vi "Do.vi"(8 "error in (no error)":errorcluster, 10 "Actor in":refnum<class "Actor.lvclass">, 11 "Self-Addressed Message":refnum<class "Self-Addressed Msg.lvclass">) -> (0 "error out":errorcluster, 2 "Actor out":refnum<class "Actor.lvclass">)   [LabVIEW 2020, in "Actor Framework.lvlib" / "Self-Addressed Msg.lvclass"]
uses:
  Self-Addressed Msg.lvclass
  Self-Addressed Msg.lvclass/Self-Addressed Msg.ctl
  Message/Message.lvclass
  Actor/Actor.lvclass
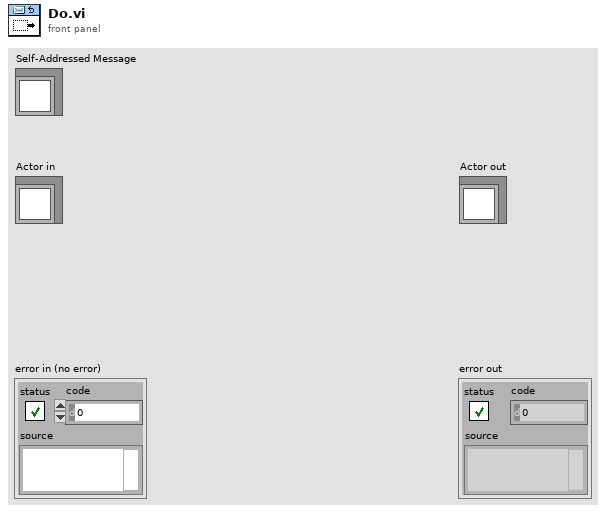
[diagram p1: front panel]
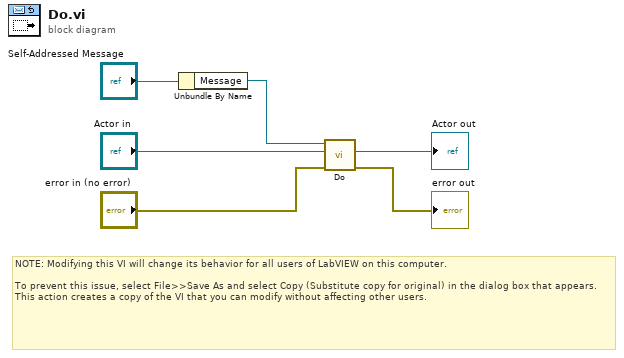
[diagram p0: block diagram]
diagram:
  # "NOTE: Modifying this VI will change its behavior for all users of LabVIEW on this computer.\n\nTo prevent this issue, select File>>Save As and select Copy (Substitute copy for original) in the dialog box that appears. This action creates a copy of the VI that you can modify without affecting other users."
  n1 = Unbundle By Name("Self-Addressed Message") -> ("Message"=w5:refnum<class "Message.lvclass">)
  n2 = call-dynamic "Do.vi"("error in (no error)"="error in (no error)", "Actor in"="Actor in", "Message"=w5) -> ("error out"=→"error out":errorcluster, "Actor out"=→"Actor out":refnum<class "Actor.lvclass">)  [unwired: 7 in]
